vi "SM8765NoiseSensor.vi"(0 "TestIndex":i32, 11 "error in":errorcluster caption="错误输入") -> (4 "返回结果":bool, 6 "dB":dbl, 15 "error out":errorcluster caption="错误输出")   [LabVIEW 2015]
uses:
  <vilib>/Instr/_visa.llb/VISA Configure Serial Port (Instr).vi
panel:
  out "COM":refnum<visa-resource-name>
  out "返回值":u8[](array[numeric]) format="%.0x"
  out "CRC16":u16 format="%.0x"
  in  "长度":u16=7
  in  "读噪声值指令":u8[](array[numeric])=[1, 3, 0, 0, 0, 1, 132, 10] format="%.0x"
  in  "延时":u32=500
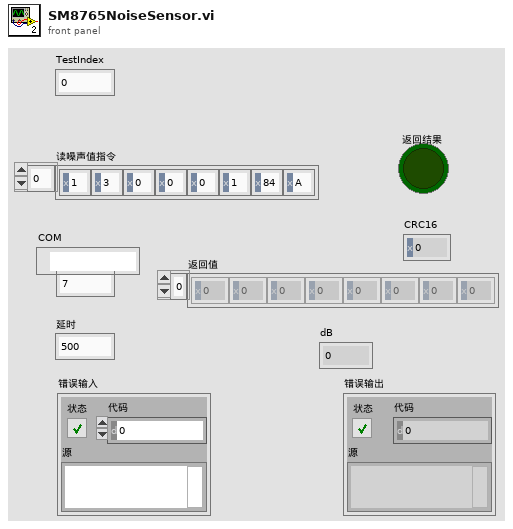
[diagram p1: front panel]
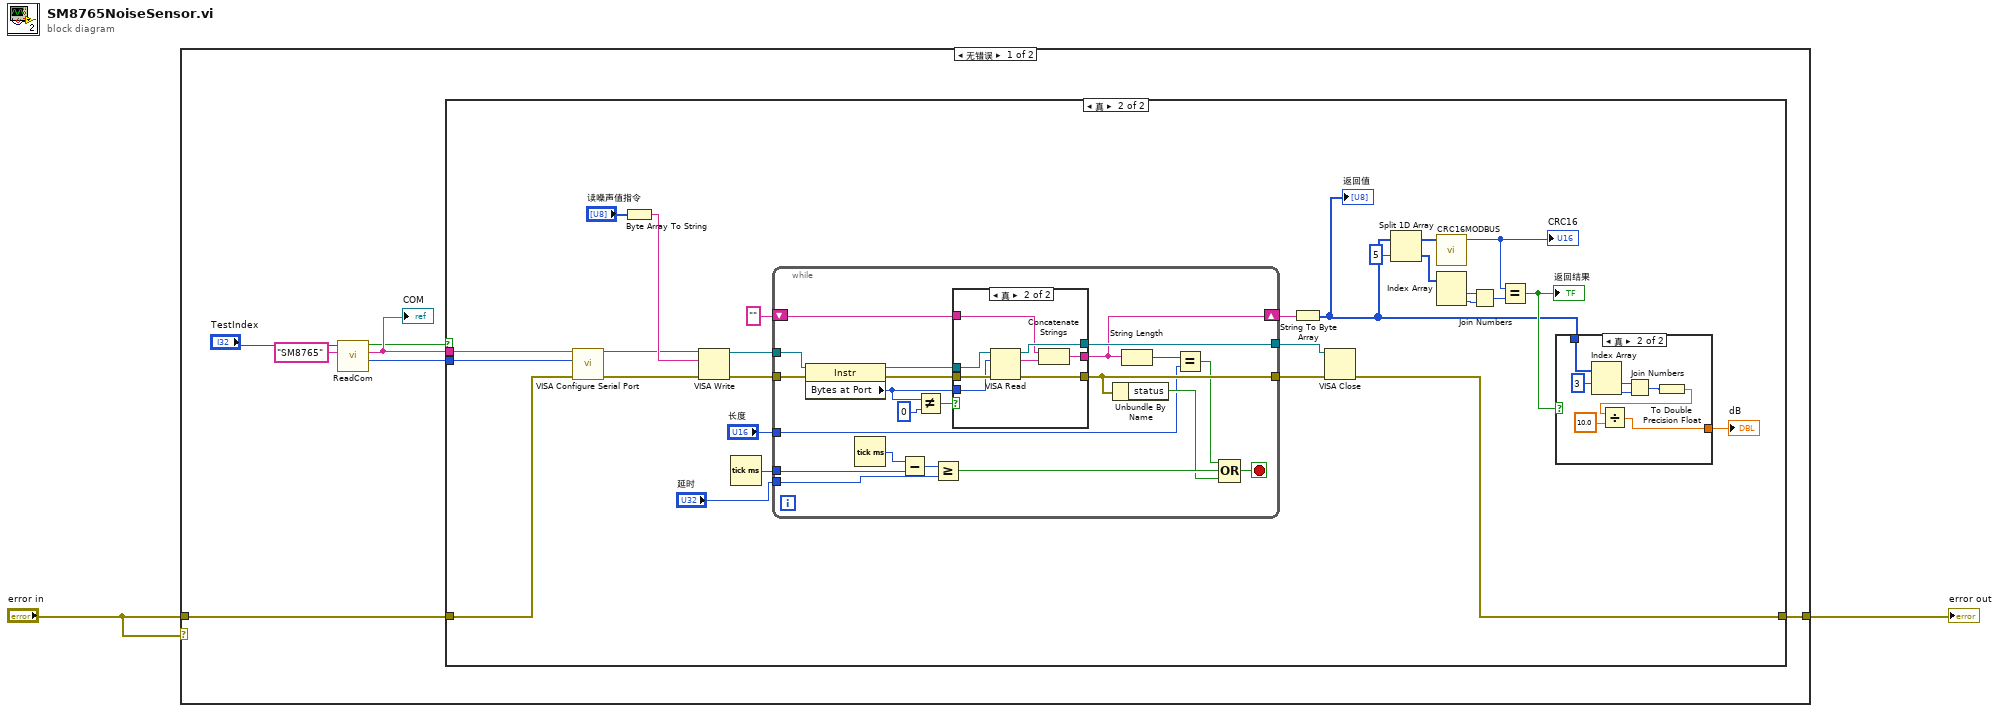
[diagram p0: block diagram]
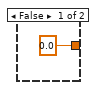
[diagram p3: hidden frame]
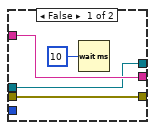
[diagram p4: hidden frame]
diagram:
  n1 = case shown="无错误" "error in" {
    tunnel: "error in" -> [w9 w80]
    tunnel: [w3 w80] -> w2
    frame No Error {
      n2 = call "ReadCom.vi"("仪器名称"="SM8765", "MyIndex"="TestIndex") -> ("Baudrate"=w4:i32, "COM"=w6:string, "OK?"=w5:bool)  [unwired: 7 in]
      "COM" <- w6
      n3 = case shown="真" w5 {
        tunnel: w9 -> [w10 w16]
        tunnel: w6 -> [_ w15]
        tunnel: w4 -> [_ w14]
        tunnel: [w10 w12] -> w3
        frame False {
        }
        frame True {
          n4 = call-poly "VISA Configure Serial Port"("VISA resource name"=w15, "baud rate (9600)"=w14, "error in (no error)"=w16) -> ("VISA resource name out"=w18:refnum<visa-resource-name>, "error out"=w17:errorcluster)  [unwired: 11 in]
          n5 = Byte Array To String(unsigned byte array="读噪声值指令") -> (string=w37:string)
          n6 = VISA Write(VISA resource name=w18, write buffer=w37, error in (no error)=w17) -> (VISA resource name out=w32:refnum<visa-resource-name>, error out=w30:errorcluster)  [unwired: 1 out]
          n7 = Tick Count (ms)() -> (millisecond timer value=w34:u32)
          n8 = while {
            tunnel: w32 -> [w66]
            tunnel: [w67] -> w11
            tunnel: w30 -> [w64]
            tunnel: [w53] -> w13
            shift-right: [w51] -> w36
            shift-left: "" ("read buffer") -> [w62]
            tunnel: w34 -> [w60]
            tunnel: "延时" -> [w57]
            tunnel: "长度" -> [w49]
            stop <- w54 stop-if-true
            n9 = property class="Instr"(reference=w66, error in=w64) -> (reference out=w65:refnum<visa-resource-name>, error out=w63:errorcluster, "Bytes at Port"=w48:u32)
            n10 = Tick Count (ms)() -> (millisecond timer value=w61:u32)
            n11 = Subtract(x=w61, y=w60) -> (x-y=w59:u32)
            n12 = Not Equal?(x=w48, y=u32 0) -> (x != y?=w55:bool)
            n13 = Greater Or Equal?(x=w59, y=w57) -> (x >= y?=w58:bool)
            n14 = case shown="真" w55 {
              tunnel: [w69 w79] -> w67
              tunnel: [w70 w78] -> w53
              tunnel: w65 -> [w69 w77]
              tunnel: w63 -> [w70 w76]
              tunnel: [w71 w74] -> w51
              tunnel: w62 -> [w71 w73]
              tunnel: w48 -> [_ w72]
              frame False {
                n15 = Wait (ms)(milliseconds to wait=u32 10 ("等待时间（毫秒）")) -> ()  [unwired: 1 out]
              }
              frame True {
                n16 = VISA Read(VISA resource name=w77, byte count=w72, error in (no error)=w76) -> (VISA resource name out=w79:refnum<visa-resource-name>, read buffer=w75:string, error out=w78:errorcluster)  [unwired: 1 out]
                n17 = Concatenate Strings(w73, w75) -> (w74:string)
              }
            }
            n18 = Unbundle By Name(w53) -> ("status"=w52:bool)
            n19 = String Length(string=w51) -> (length=w50:i32)
            n20 = Equal?(x=w50, y=w49) -> (x = y?=w47:bool)
            n21 = Compound Arithmetic op=OR ("复合运算")(w47, w58, w52) -> (w54:bool)
          }
          n22 = String To Byte Array(string=w36) -> (unsigned byte array=w20:u8[])
          "返回值" <- w20
          n23 = VISA Close(VISA resource name=w11, error in (no error)=w13) -> (error out=w12:errorcluster)
          n24 = Split 1D Array(array=w20, index=5 ("索引")) -> (first subarray=w27:u8[], second subarray=w26:u8[])
          n25 = call "CRC16MODBUS.vi"("In_Data"=w27) -> ("CRC16"=w23:u16)  [unwired: 9 in, 1 out]
          "CRC16" <- w23
          n26 = Index Array(array=w26) -> (element #1=w24:u8, element #2=w25:u8)  [unwired: 2 in]
          n27 = Join Numbers(hi=w24, lo=w25) -> ((hi.lo)=w22:u16)
          n28 = Equal?(x=w23, y=w22) -> (x = y?=w21:bool)
          "返回结果" <- w21
          n29 = case shown="真" w21 {
            tunnel: w20 -> [_ w46]
            tunnel: [0.0 w39] -> w19
            frame False {
            }
            frame True {
              n30 = Index Array(array=w46, index #1=3 ("索引")) -> (element #1=w44:u8, element #2=w43:u8)  [unwired: 1 in]
              n31 = Join Numbers(hi=w44, lo=w43) -> ((hi.lo)=w41:u16)
              n32 = To Double Precision Float(number=w41) -> (double precision float=w40:dbl)
              n33 = Divide(x=w40, y=10.0) -> (x/y=w39:dbl)
            }
          }
          "dB" <- w19
        }
      }
    }
    frame Error {
    }
  }
  "error out" <- w2
